vi "StdObjectArray_get_and_lock.vi"(8 "error in (no error)":errorcluster) -> (0 "error out":errorcluster, 3 "StandardObjects":refnum<class "Standard.lvclass">[](array[class]))   [LabVIEW 2018]
doc: "the VI locks and returns/reads the StandardObjectsArray using a Queue"
uses:
  Classes/Standard/Standard.lvclass
  global variables.vi
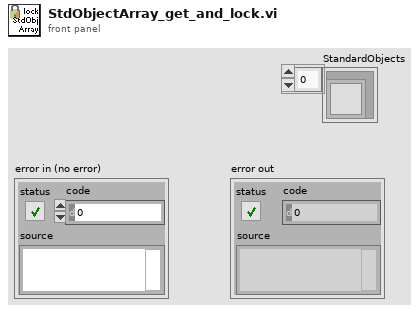
[diagram p1: front panel]
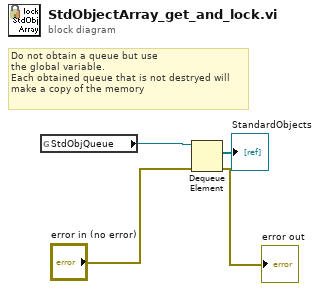
[diagram p0: block diagram]
diagram:
  # "Do not obtain a queue but use\nthe global variable.\nEach obtained queue that is not destryed will\nmake a copy of the memory"
  n1 = global read "global variables.vi" "StdObjQueue"() -> (w3:refnum<queue>)
  n2 = Dequeue Element(queue=w3, error in (no error)="error in (no error)") -> (element=→"StandardObjects":refnum<class "Standard.lvclass">[], error out=→"error out":errorcluster)  [unwired: 1 in, 2 out]
